vi "localeSystemDecimalDot (SubVI).vi"() -> (1 "InvlocaleSystemDecimal":string, 2 "localeSystemDecimal":string, 3 "localeSystemDecimalDot":bool)   [LabVIEW 2017, in "LV_Unicorn.lvlib"]
uses:
  LV_Unicorn.lvlib
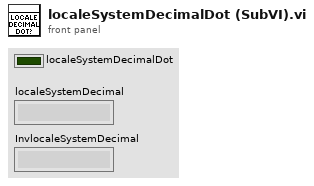
[diagram p1: front panel]
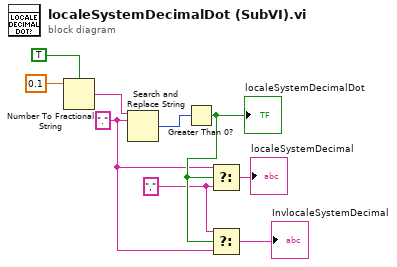
[diagram p0: block diagram]
diagram:
  w3 = "," ("f")
  w2 = "." ("search string")
  n1 = Number To Fractional String(use system decimal point (T)=TRUE, number=0.1) -> (F-format string=w8:string)  [unwired: 2 in]
  n2 = Search and Replace String(input string=w8, search string=w2) -> (number of replacements=w9:i32)  [unwired: 6 in, 3 out]
  n3 = Greater Than 0?(x=w9) -> (x > 0?=w4:bool)
  "localeSystemDecimalDot" <- w4
  n4 = Select(t=w2, s=w4, f=w3) -> (s? t:f=→"localeSystemDecimal":string)
  n5 = Select(t=w3, s=w4, f=w2) -> (s? t:f=→"InvlocaleSystemDecimal":string)
